vi "CNT Stop Counter.vi"(9 "Channel":u8, 10 "DevIndex":i32, 11 "DevType":i32) -> (3 "function return":i32)   [LabVIEW 2010, in "ControlCNT.lvlib"]
doc: "int WINAPI CNT_StopCounter(int DevType, int DevIndex, unsigned char Channel);"
uses:
  ControlCNT.lvlib
  ControlCNT/Ginkgo_Driver.dll
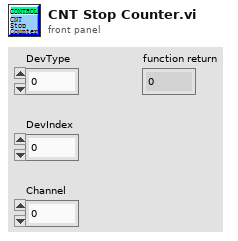
[diagram p1: front panel]
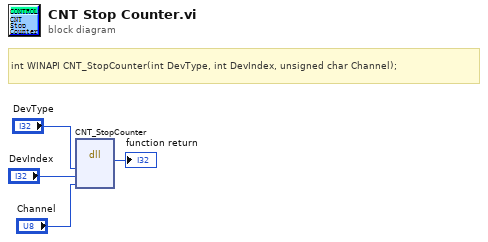
[diagram p0: block diagram]
diagram:
  # "int WINAPI CNT_StopCounter(int DevType, int DevIndex, unsigned char Channel);"
  n1 = dll-call lib="E:/Project/vt_ginkgo/truck/Ginkgo Driver/vs2010/Ginkgo_USB-I2C&SPI&CAN_API_v2.0.3.3/lib/labview_32bit/ControlCNT/Ginkgo_Driver.*" fn="CNT_StopCounter"("DevType"="DevType", "DevIndex"="DevIndex", "Channel"="Channel") -> (→"function return":i32)  [unwired: 6 in, 2 out]
